vi "Query Assets.vi"() -> ()   [LabVIEW 2019]
uses:
  <vilib>/Skyline/Configuration/Configuration HTTP_class/NI Skyline Configuration HTTP.lvclass/NI Skyline Configuration HTTP.ctl
  <vilib>/Skyline/Configuration/Configuration HTTP_class/Open Configuration HTTP Auto.vi
  <vilib>/Skyline/Configuration/Configuration HTTP_class/Read Server URL.vi
  <vilib>/Skyline/Configuration/HTTP/Open Configuration Auto (Custom).vi
  <vilib>/Skyline/Configuration/HTTP/Configuration File Cache.vi
  <vilib>/Skyline/Configuration/HTTP/Initialize From Auto Configuration.vi
  <vilib>/httpClient/POSTBuffer.vi
  <vilib>/Skyline/Configuration/Configuration HTTP_class/NI Skyline Configuration HTTP.lvclass
  <vilib>/Skyline/Configuration/Configuration_class/NI Skyline Configuration.lvclass
  <vilib>/httpClient/LabVIEWHTTPClient.lvlib
  <vilib>/Skyline/Utilities/NI Skyline Utilities.lvlib
panel:
  out "body":string
  out "Server URL":string
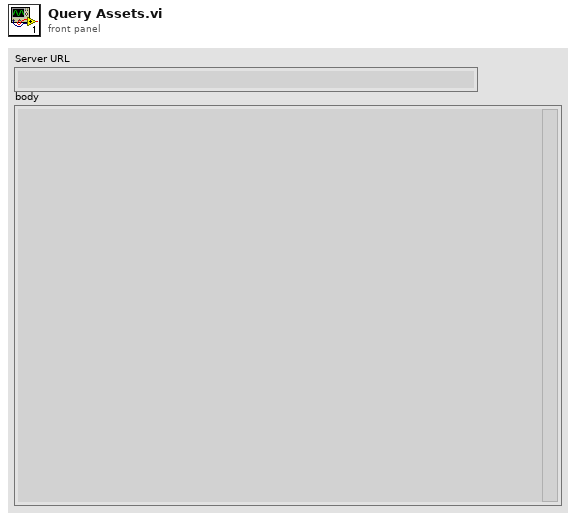
[diagram p1: front panel]
types:
  T1 = typedef "LabVIEWHTTPClient.lvlib/ClientHandle.ctl" = refnum<k1>
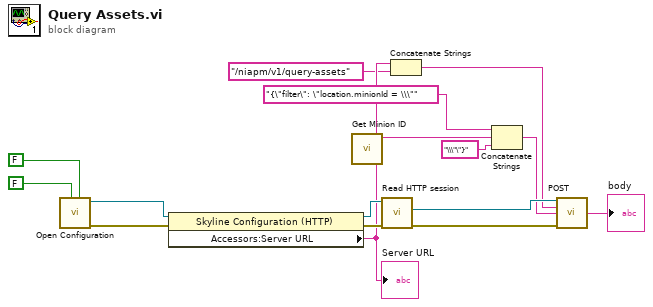
[diagram p0: block diagram]
diagram:
  n1 = call-poly <vilib>:"Open Configuration.vi"("HTTPS only?"=FALSE, "verify server?"=FALSE) -> ("error out"=w12:errorcluster, "configuration"=w13:refnum<class "NI Skyline Configuration HTTP.lvclass">)  [unwired: 8 in]
  n2 = property class="Skyline Configuration (HTTP)"(reference=w13, error in=w12) -> (reference out=w11:refnum<class "NI Skyline Configuration HTTP.lvclass">, error out=w10:errorcluster, "Accessors:Server URL"=w8:string)
  "Server URL" <- w8
  n3 = call <vilib>:"Get Minion ID.vi"() -> ("minion id"=w3:string)  [unwired: 11 in]
  n4 = call <vilib>:"Read HTTP session.vi"("error in (no error)"=w10, "HTTP configuration in"=w11) -> ("error out"=w9:errorcluster, "http session"=w14:T1)  [unwired: 7 in, 1 out]
  n5 = Concatenate Strings(w8, "/niapm/v1/query-assets" ("string")) -> (w7:string)
  n6 = Concatenate Strings("{\"filter\": \"location.minionId = \\\"" ("buffer"), w3, "\\\"\"}" ("buffer")) -> (w1:string)
  n7 = call-poly <vilib>:"POST.vi"("client handle"=w14, "url"=w7, "buffer"=w1, "error in (no error)"=w9) -> ("body"=→"body":string)  [unwired: 8 in, 3 out]
